vi "Get Surface Color Map.vi"(9 "Levels":sgl=255.0, 11 "Amplifiy":sgl[](array[numeric])) -> (3 "Color Index Array":i32[](array[numeric]))   [LabVIEW 2020, in "3D Plot Datatype.lvclass"]
uses:
  <vilib>/Math Plots/3D Math Plots/3D Plot/3D Plot Datatype/3D Plot Datatype.lvclass
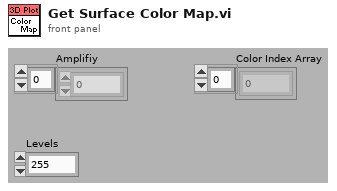
[diagram p1: front panel]
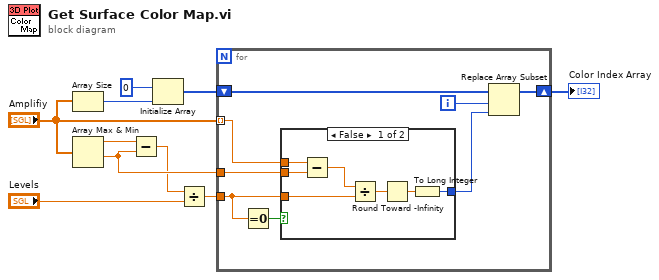
[diagram p0: block diagram]
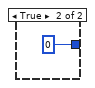
[diagram p2: hidden frame]
diagram:
  n1 = Array Size(array="Amplifiy") -> (size(s)=w1:i32)
  n2 = Array Max & Min(array="Amplifiy") -> (max value=w5:sgl, min value=w8:sgl)  [unwired: 2 out]
  n3 = Subtract(x=w5, y=w8) -> (x-y=w6:sgl)
  n4 = Initialize Array(0, w1) -> (w3:i32[])
  n5 = Divide(x=w6, y="Levels") -> (x/y=w9:sgl)
  n6 = for {
    tunnel: "Amplifiy" -> [w18] mode=indexing
    tunnel: w8 -> [w17]
    tunnel: w9 -> [w12]
    shift-right: [w16] -> w10
    shift-left: w3 -> [w15]
    i -> [w13]
    n7 = Equal To 0?(x=w12) -> (x = 0?=w11:bool)
    n8 = case shown="False" w11 {
      tunnel: w18 -> [w25 _]
      tunnel: w17 -> [w24 _]
      tunnel: [w20 0] -> w14
      tunnel: w12 -> [w19 _]
      frame False {
        n9 = Subtract(x=w25, y=w24) -> (x-y=w23:sgl)
        n10 = Divide(x=w23, y=w19) -> (x/y=w21:sgl)
        n11 = Round Toward -Infinity(1:w21) -> (0:w22:sgl)
        n12 = To Long Integer(number=w22) -> (32bit integer=w20:i32)
      }
      frame True {
      }
    }
    n13 = Replace Array Subset(array=w15, new element=w14, index=w13) -> (w16:i32[])
  }
  "Color Index Array" <- w10
